vi "CC FITS Write DEC Header.vi"(10 "Detector #":u16, 11 "HK Channel":refnum<class "HK Table.lvclass">) -> (2 "DEC out":dbl, 3 "RA out":dbl)   [LabVIEW 2021]
uses:
  hk-channel-class/HK Table/HK Table.lvclass
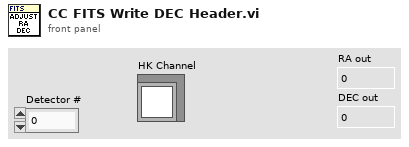
[diagram p1: front panel]
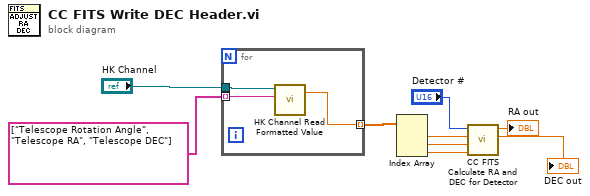
[diagram p0: block diagram]
diagram:
  n1 = for {
    tunnel: string[] ["Telescope Rotation Angle", "Telescope RA", "Telescope DEC"] -> [w12] mode=indexing
    tunnel: "HK Channel" -> [w11]
    tunnel: [w10] -> w7 mode=indexing
    n2 = call-dynamic "HK Channel Read Formatted Value.vi"("Name"=w12, "HK Channel in"=w11) -> ("Value"=w10:dbl)  [unwired: 2 in, 7 out]
  }
  n3 = Index Array(array=w7) -> (element #1=w6:dbl, element #2=w4:dbl, element #3=w3:dbl)  [unwired: 3 in]
  n4 = call "CC FITS Calculate RA and DEC for Detector.vi"("DEC"=w3, "RA"=w4, "ROT"=w6, "Detector #"="Detector #") -> ("DEC out"=→"DEC out":dbl, "RA out"=→"RA out":dbl)  [unwired: 6 in]
